vi "Get Enum Getters.vi"(8 "error in (no error)":errorcluster, 11 "enum ref in":refnum<vi>) -> (0 "error out":errorcluster, 2 "enum strings":string[](array[string]), 3 "enum numbers":i32[](array[numeric]))   [LabVIEW 2020, in "MeasurementServerTests.lvlib"]
uses:
  MeasurementServerTests.lvlib
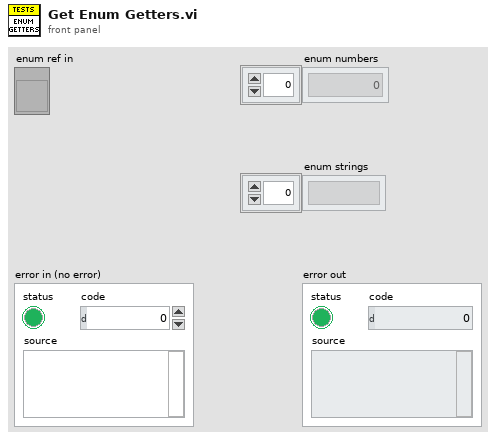
[diagram p1: front panel]
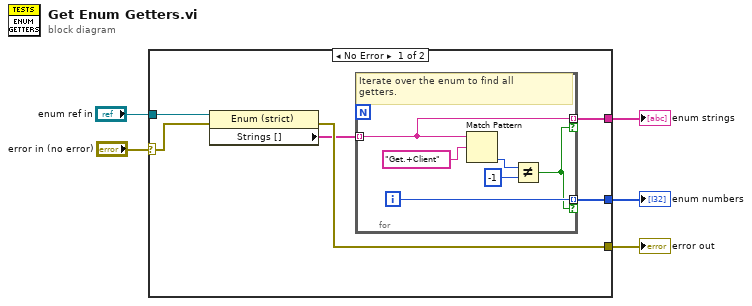
[diagram p0: block diagram]
diagram:
  n1 = case shown="No Error" "error in (no error)" {
    selector: "error in (no error)" -> [w9 w18]
    tunnel: [w11 _] -> w5
    tunnel: [w10 w18] -> w4
    tunnel: [w8 _] -> w2
    tunnel: "enum ref in" -> [w6 _]
    frame No Error {
      n2 = property on="Property Node" class="Enum (strict)"(reference=w6, error in=w9) -> (error out=w10:errorcluster, "Strings []"=w7:string[])  [unwired: 1 out]
      n3 = for {
        tunnel: w7 -> [w13] mode=indexing
        tunnel: [w14] -> w8 mode=indexing if=w12
        tunnel: [w13] -> w11 mode=indexing if=w12
        i -> [w14]
        # "Iterate over the enum to find all\ngetters."
        n4 = Match Pattern(string=w13, regular expression="Get.+Client") -> (offset past match=w16:i32)  [unwired: 1 in, 3 out]
        n5 = Not Equal?(x=w16, y=-1) -> (x != y?=w12:bool)
      }
    }
    frame Error {
    }
  }
  "enum strings" <- w5
  "error out" <- w4
  "enum numbers" <- w2
